vi "Datum_Image_Calibration.vi"(3 "Mode":T11=enum."Run VI", 5 "Traverse line In":T8={"Start X"=1950.0, "Start Y"=0.0, "Start Z"=250.0, "End X"=nan, "End Y"=nan, "End Z"=nan, "No. of pts."=0, "Spacing"=enum."N/A", "Filename"=path "C:/Enflo_Data_Local/2016/EnFlo_Tunnel/Paul_Hayden/Calibrations/Cal_03-2016/50mm_Y_Strip.xls", "Tunnel Speed"=nan, "Averaging time (min)"=nan, "Extra Commands"="", "Carrier_1 Q (l/min)"=nan, "Carrier_2 Q (l/min)"=nan, "Trace Gas Concentration (%)"=nan, "Specific Arguments"="Datum_Image_Calibration.vi; X Fixed", "Comments"="", "Row No"=0, "Row Type Selector"=enum."Run VI Named:", "Completion time"="12:00  22-03-2016", "Row Duration (mins)"=0.08333333333333333, "No. of Valid pts."=0, "Meas Setup File"="Trav_Cam_Picture.xls"} {"Carrier_2 Q (l/min)" format="%#.2f"; "Row Duration (mins)" format="%#.1f"; "Row No" min=0; "Trace Gas Concentration (%)" min=0.0 format="%#_4f"; "Carrier_1 Q (l/min)" format="%#.2f"; "Tunnel Speed" format="%#.2f"; "Start X" format="%#.2f"; "Start Y" format="%#.2f"; "Start Z" format="%#.2f"; "End X" format="%#.2f"; "End Y" format="%#.2f"; "End Z" format="%#.2f"; "Averaging time (min)" min=0.0 format="%#.2f"}) -> (0 "Error Message":string, 1 "Status":T7, 2 "Traverse line Out":T8={"Start X"=1950.0, "Start Y"=0.0, "Start Z"=250.0, "End X"=nan, "End Y"=nan, "End Z"=nan, "No. of pts."=0, "Spacing"=enum."N/A", "Filename"=path "C:/Enflo_Data_Local/2016/EnFlo_Tunnel/Paul_Hayden/Calibrations/Cal_03-2016/50mm_Y_Strip.xls", "Tunnel Speed"=nan, "Averaging time (min)"=nan, "Extra Commands"="", "Carrier_1 Q (l/min)"=nan, "Carrier_2 Q (l/min)"=nan, "Trace Gas Concentration (%)"=nan, "Specific Arguments"="Datum_Image_Calibration.vi; X Fixed", "Comments"="", "Row No"=0, "Row Type Selector"=enum."Run VI Named:", "Completion time"="12:00  22-03-2016", "Row Duration (mins)"=0.08333333333333333, "No. of Valid pts."=0, "Meas Setup File"="Trav_Cam_Picture.xls"} {"Carrier_2 Q (l/min)" format="%#.2f"; "Row Duration (mins)" format="%#.1f"; "Row No" min=0; "Trace Gas Concentration (%)" min=0.0 format="%#_4f"; "Carrier_1 Q (l/min)" format="%#.2f"; "Tunnel Speed" format="%#.2f"; "Start X" format="%#.2f"; "Start Y" format="%#.2f"; "Start Z" format="%#.2f"; "End X" format="%#.2f"; "End Y" format="%#.2f"; "End Z" format="%#.2f"; "Averaging time (min)" min=0.0 format="%#.2f"})   [LabVIEW 2015]
uses:
  Gen Trav/Traverse_cluster.ctl
  Gen Trav/Spacing.ctl
  Controls/Multi_run_mode.ctl
  Controls/User_Specific_mode.ctl
  Gen Trav/Multi_Run_Status.ctl
  Utilities/Image acquisition and processing/Feature detection/Typedefs/ROI bounds.ctl
  Utilities/Image acquisition and processing/Feature detection/Typedefs/Theta range.ctl
  Camera Server/Camera enum/Camera enum.ctl
  Utilities/Image acquisition and processing/Feature detection/Typedefs/Txy range.ctl
  Utilities/Image acquisition and processing/Feature detection/Typedefs/Top level controls.ctl
  Camera Server/Camera enum/Camera resolution.ctl
  Gen Trav/Status_Cluster.ctl
  <vilib>/Analysis/baseanly.llb/Mean (DBL).vi
  Globals/Constants_global.vi
  <vilib>/Analysis/NI_AALBase.lvlib
panel:
  in  "Resolution":T1=2 items=["Low", "Med.", "High", "Max."]
  out "Setup file?":bool
  in  "Controls":T2={"Auto ROI (for rot.)"=FALSE, "Apply scaling"=FALSE, "Apply rotation"=TRUE, "Apply Tx"=FALSE, "Apply Ty"=FALSE, "Keep proc. img"=FALSE}
  in  "Txy range (pixels)":T3={"Tx max (pix)"=150, "Tx min (pix)"=-150, "Ty max (pix)"=10, "Ty min (pix)"=-10}
  in  "Quality":u32=750 max=1000
  in  "Camera":T4="Travcam"
  in  "Theta range (deg)":T5={"theta max (deg)"=20.0, "theta min (deg)"=-20.0}
  in  "ROI to crop (pixels)":T6={"Xmax"=458, "Ymax"=346, "Xmin"=252, "Ymin"=131}
  out "Scale":dbl[](graph)
  out "Angle":dbl[](graph)=[-89.79324776154536, -89.74497086066056, -89.6724887953992, -89.66762827818829]
  out "Displacments":sgl[][](array[numeric])=[[-0.0, -0.0], [-0.0, -5.0], [-0.0, -10.0], [-0.0, 5.0], [-0.0, 10.0]]
  in  "Averaging time (s) (from end)":dbl=1.0
  in  "Duration (s)":dbl=5.0
  # "X           Y            Z"
  # "Start"
  # "End"
  # "X           Y            Z"
  # "Start"
  # "End"
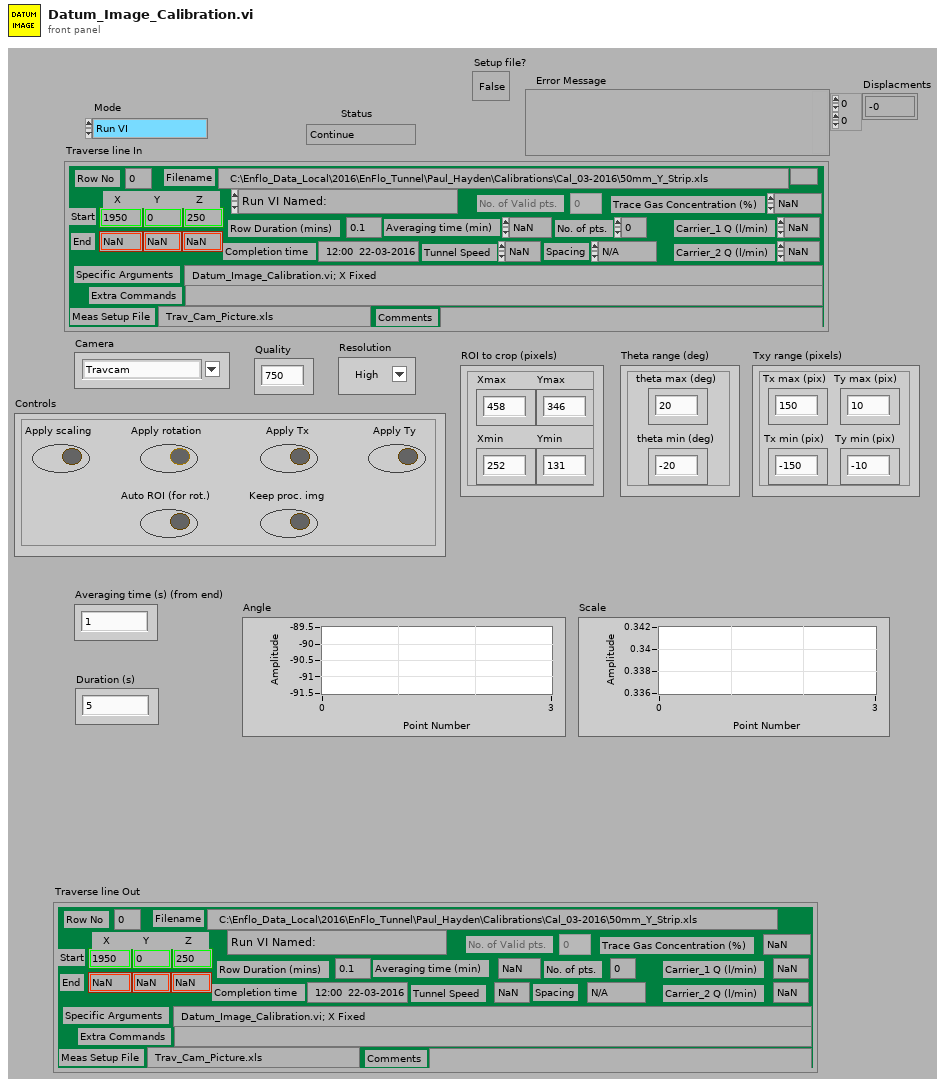
[diagram p1: front panel]
types:
  T1 = typedef "Camera resolution.ctl" = u8
  T2 = typedef "Top level controls.ctl" = cluster{"Auto ROI (for rot.)":bool, "Apply scaling":bool, "Apply rotation":bool, "Apply Tx":bool, "Apply Ty":bool, "Keep proc. img":bool}
  T3 = typedef "Txy range.ctl" = cluster{"Tx max (pix)":i32, "Tx min (pix)":i32, "Ty max (pix)":i32, "Ty min (pix)":i32}
  T4 = typedef "Camera enum.ctl" = string
  T5 = typedef "Theta range.ctl" = cluster{"theta max (deg)":dbl, "theta min (deg)":dbl}
  T6 = typedef "ROI bounds.ctl" = cluster{"Xmax":i32, "Ymax":i32, "Xmin":i32, "Ymin":i32}
  T7 = typedef "Multi_Run_Status.ctl" = enum16{"Continue", "Jump to Next Point", "Jump to Next Row", "Jump To Fall Back", "Terminate Run"}
  T8 = typedef "Traverse_cluster.ctl" = cluster{"Start X":sgl, "Start Y":sgl, "Start Z":sgl, "End X":sgl, "End Y":sgl, "End Z":sgl, "No. of pts.":i32, "Spacing":T9, "Filename":path, "Tunnel Speed":dbl, "Averaging time (min)":dbl, "Extra Commands":string, "Carrier_1 Q (l/min)":dbl, "Carrier_2 Q (l/min)":dbl, "Trace Gas Concentration (%)":dbl, "Specific Arguments":string, "Comments":string, "Row No":i32, "Row Type Selector":T10, "Completion time":string, "Row Duration (mins)":dbl, "No. of Valid pts.":i32, "Meas Setup File":string}
  T9 = typedef "Spacing.ctl" = enum16{"Linear", "Log", "Gauss", "Specified", "N/A"}
  T10 = typedef "Multi_run_mode.ctl" = enum16{"Move Traverse Only", "Set Tunnel Speed Only", "Set Source Only", "Set Measurement Conditions", "Single Measurement", "Vertical Profile", "Lateral Profile", "Longitudinal Profile", "Explore Volume", "Multi-Axis Profile", "Auto Calibrate", "Meas Fast FID Bkgnd", "Check Beam Power", "Scanning Valve Measurement", "Run VI Named:", "Set ADAM Ch", "Wait (minutes)", "Send Message", "Synchronize With:", "Fall Back to this Row", "Turn Off Row Repeating", "Blank Row", "Traverse 3D Volume"}
  T11 = typedef "User_Specific_mode.ctl" = enum16{"Check VI only", "Run VI"}
  T12 = typedef "Status_Cluster.ctl" = cluster{"Status":T7, "Error Type":string, "Error Description":string}
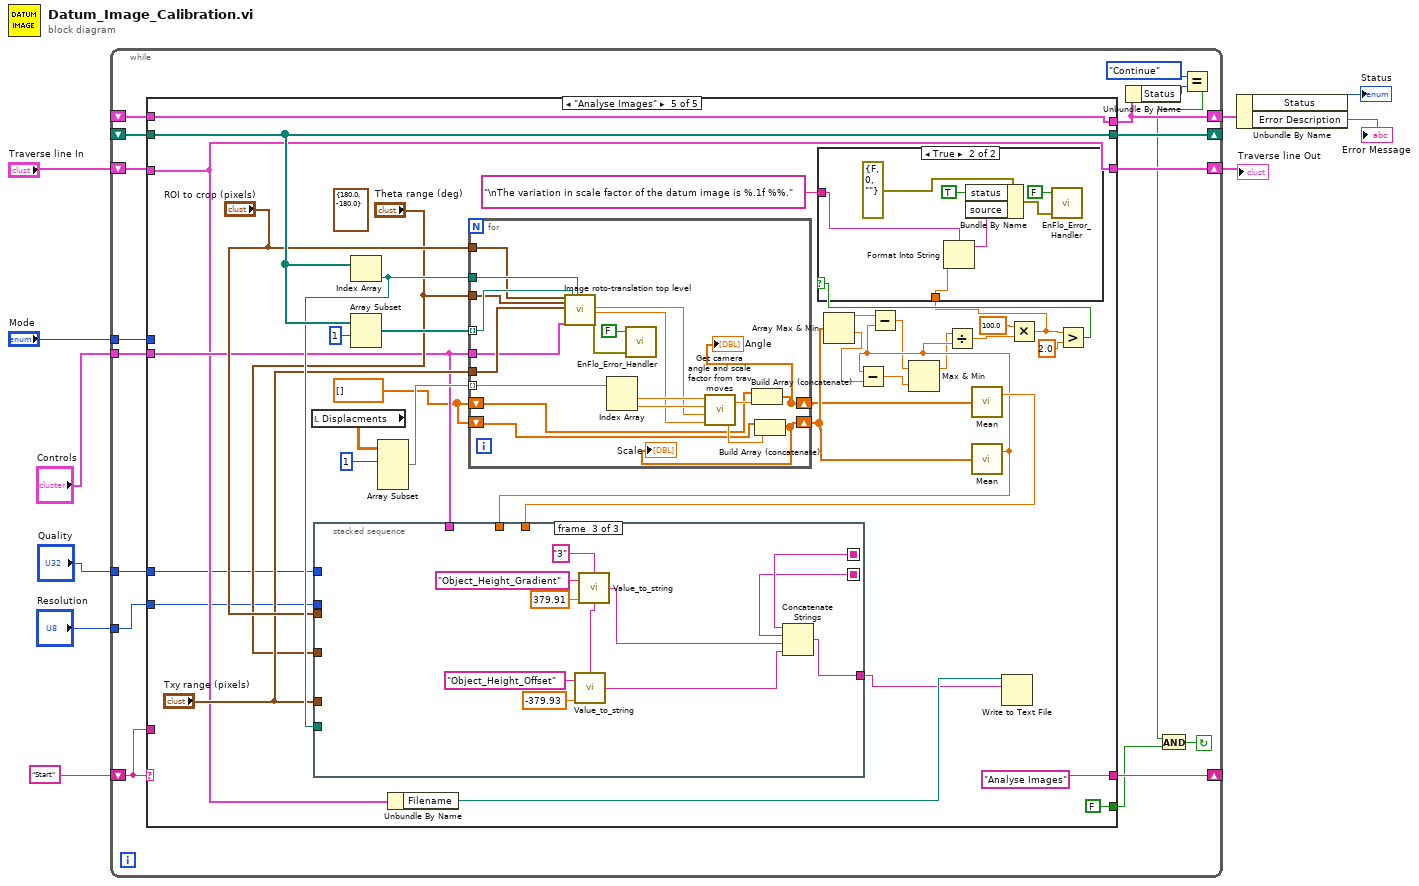
[diagram p0: block diagram]
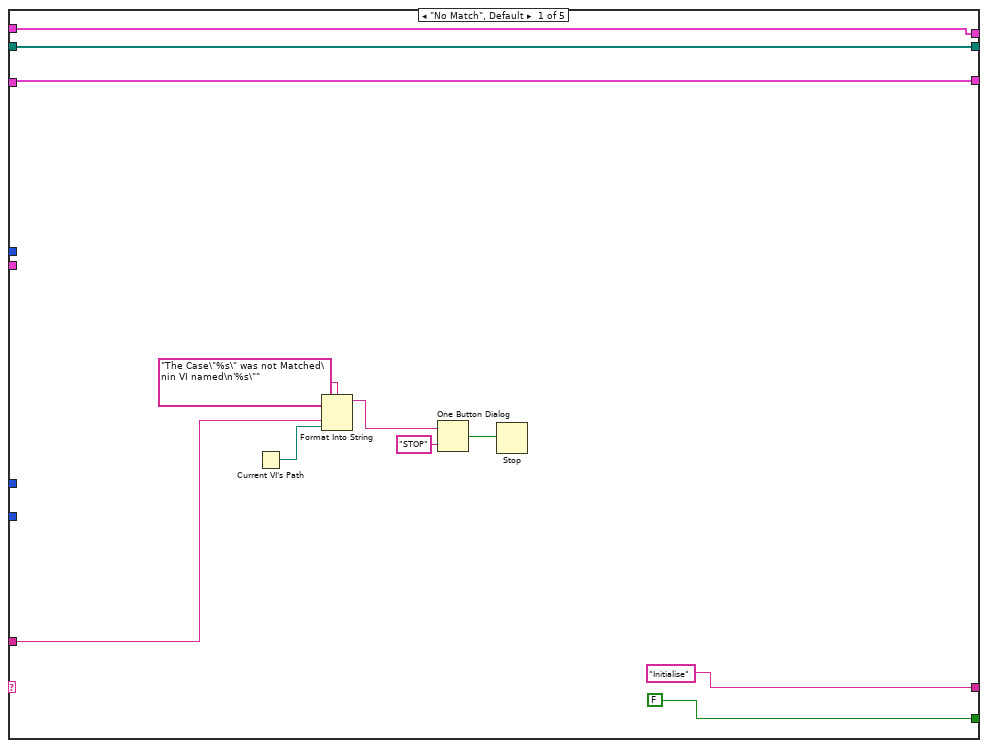
[diagram p2: hidden frame]
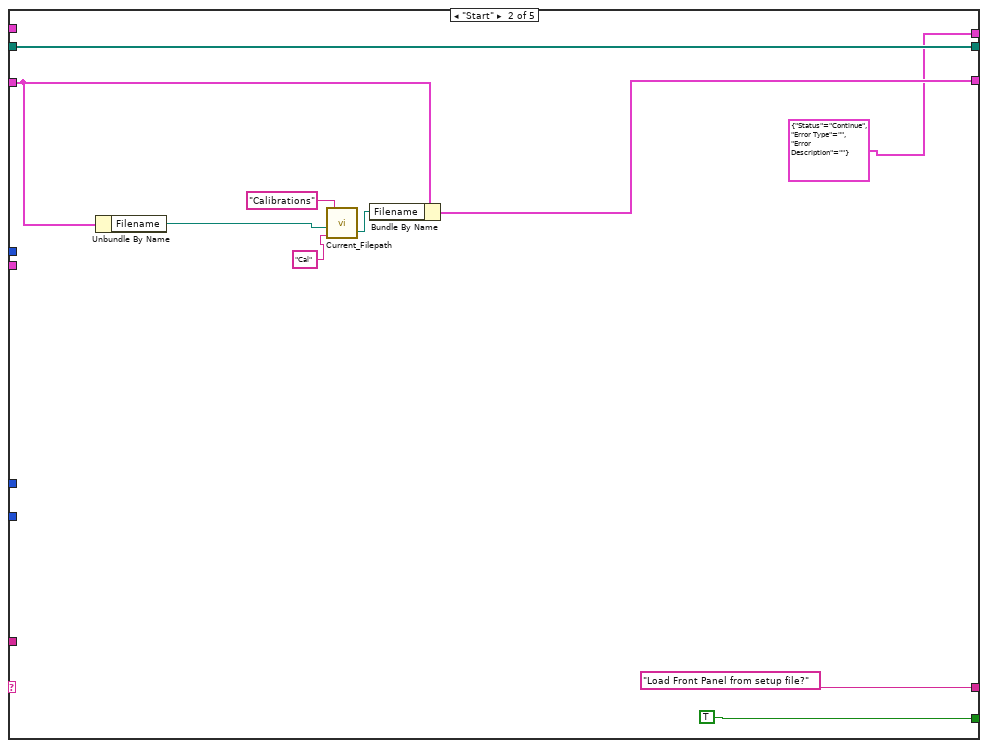
[diagram p3: hidden frame]
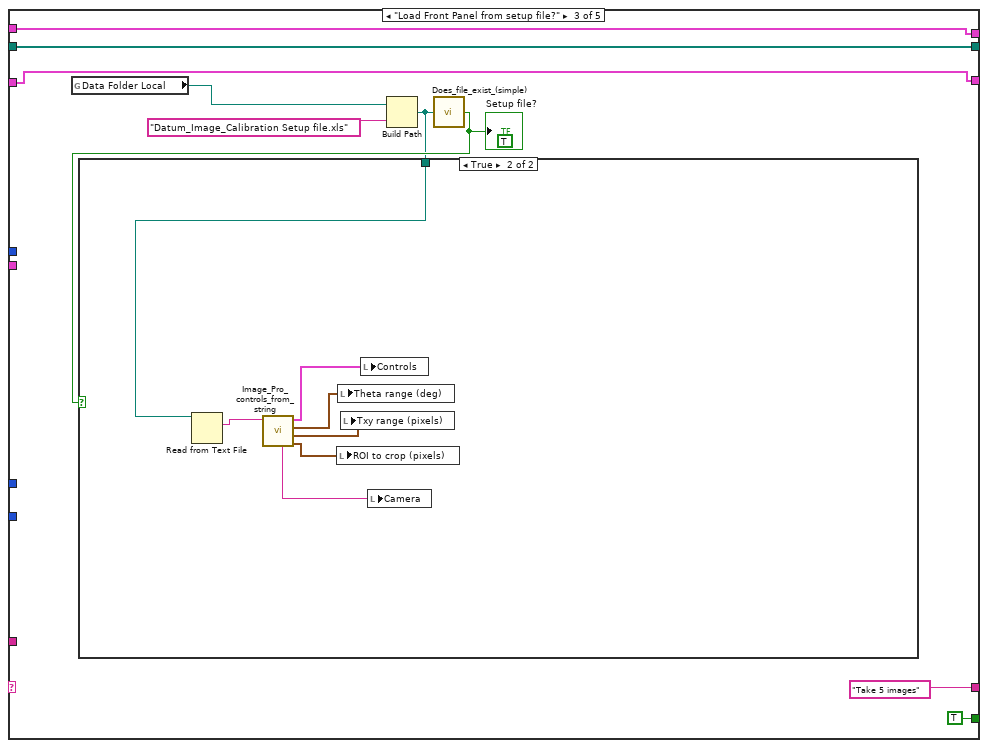
[diagram p4: hidden frame]
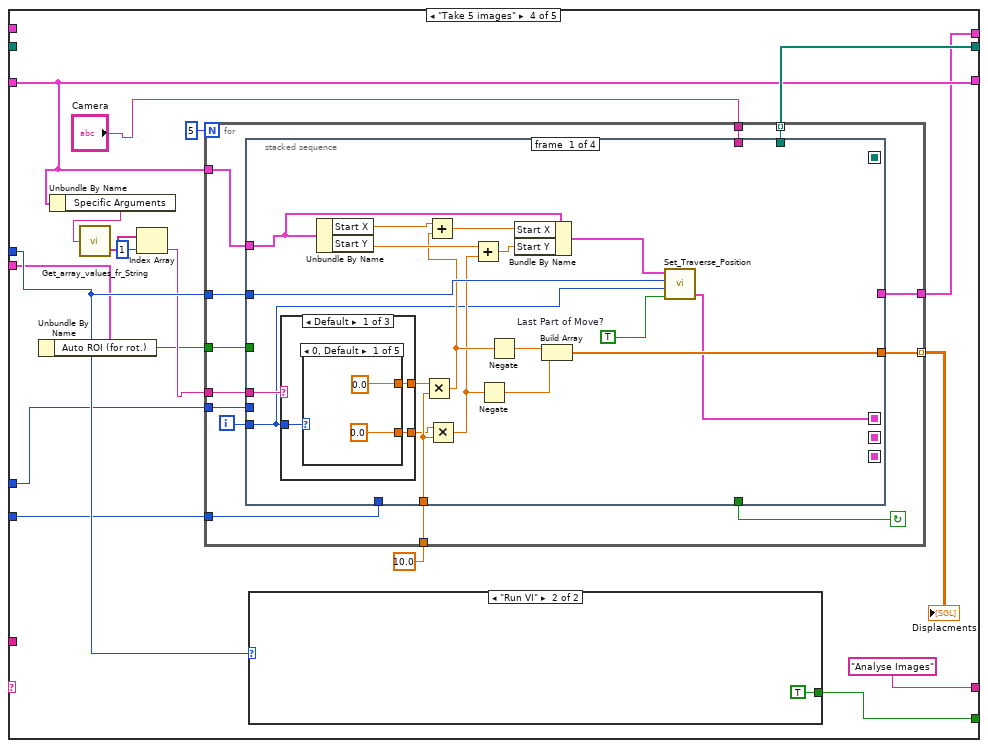
[diagram p6: hidden frame]
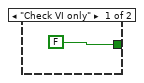
[diagram p7: hidden frame]
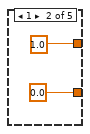
[diagram p8: hidden frame]
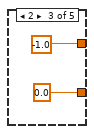
[diagram p9: hidden frame]
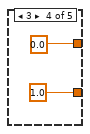
[diagram p10: hidden frame]
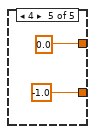
[diagram p11: hidden frame]
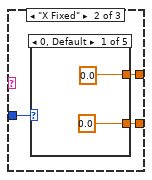
[diagram p12: hidden frame]
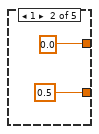
[diagram p13: hidden frame]
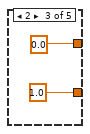
[diagram p14: hidden frame]
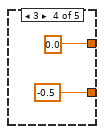
[diagram p15: hidden frame]
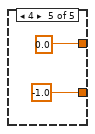
[diagram p16: hidden frame]
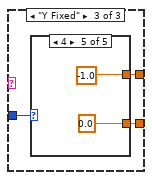
[diagram p17: hidden frame]
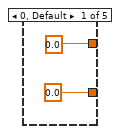
[diagram p18: hidden frame]
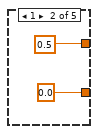
[diagram p19: hidden frame]
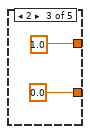
[diagram p20: hidden frame]
diagram:
  n1 = while {
    shift-left: "Start" -> [w26]
    shift-right: [w27] -> _
    tunnel: "Mode" -> [w25]
    shift-right: [w23] -> w7
    shift-left: "Traverse line In" -> [w24]
    shift-right: [w22] -> _
    shift-left: _ -> [w21]
    tunnel: "Controls" -> [w20]
    shift-right: [w19] -> w5
    shift-left: _ -> [w13]
    tunnel: "Quality" -> [w12]
    tunnel: "Resolution" -> [w11]
    stop <- w15 continue-if-true
    n2 = case shown="\"Analyse Images\"" w26 {
      tunnel: [FALSE TRUE TRUE w77 FALSE] -> w16
      tunnel: ["Initialise" "Load Front Panel from setup file?" "Take 5 images" "Analyse Images" "Analyse Images"] -> w27
      tunnel: w26 -> [w33 _ _ _ _]
      tunnel: w25 -> [_ _ _ w78 _]
      tunnel: w24 -> [w30 w43 w50 w70 w225]
      tunnel: [w30 w42 w50 w70 w225] -> w23
      tunnel: [w29 w41 w51 w79 w241] -> w22
      tunnel: w21 -> [w29 w41 w51 _ w241]
      tunnel: w20 -> [_ _ _ w67 w228]
      tunnel: [w28 T12 {"Status"=enum."Continue", "Error Type"="", "Error Description"=""} ("Status Cluster Out") w49 w69 w210] -> w19
      tunnel: w13 -> [w28 _ w49 _ w210]
      tunnel: w12 -> [_ _ _ w68 w211]
      tunnel: w11 -> [_ _ _ w65 w209]
      frame "No Match", Default {
        n3 = Current VI's Path() -> (path=w32:path)
        n4 = Format Into String(format string="The Case\"%s\" was not Matched\nin VI named\n'%s\"" ("Format String"), w33, w32) -> (resulting string=w36:string)  [unwired: 2 in, 1 out]
        n5 = One Button Dialog(message=w36, button name ("OK")="STOP") -> (true=w34:bool)
        n6 = Stop(stop? (T)=w34) -> ()
      }
      frame "Start" {
        n7 = Unbundle By Name(w43) -> ("Filename"=w45:path)
        n8 = call "Current_Filepath.vi"("Short_Name"="Cal" ("Data Type"), "Filename in"=w45, "Data Type"="Calibrations") -> ("Filename Out"=w40:path)  [unwired: 1 in, 1 out]
        n9 = Bundle By Name(cluster=w43, "Filename"=w40) -> (w42:T8)
      }
      frame "Load Front Panel from setup file?" {
        (unwired) TRUE ("exists?")
        n10 = global read "Constants_global.vi" "Data Folder Local"() -> (w55:path)
        n11 = Build Path(base path=w55, name or relative path="Datum_Image_Calibration Setup file.xls") -> (appended path=w52:path)
        n12 = call "Does_file_exist_(simple).vi"("Pathname"=w52) -> ("exists?"=w53:bool)
        "Setup file?" <- w53
        n13 = case shown="True" w53 {
          tunnel: w52 -> [_ w64]
          frame False {
          }
          frame True {
            n14 = Read from Text File(file (use dialog)=w64) -> (text=w63:string)  [unwired: 3 in, 3 out]
            n15 = call "Image_Pro_controls_from_string.vi"("Setup String"=w63) -> ("ROI to crop (pixels)"=w59:T6, "Txy range (pixels)"=w60:T3, "Theta range (deg)"=w61:T5, "Controls"=w62:T2, "Camera"=w58:string)  [unwired: 4 in, 2 out]
            n16 = local write "ROI to crop (pixels)"(w59) -> ()
            n17 = local write "Theta range (deg)"(w61) -> ()
            n18 = local write "Txy range (pixels)"(w60) -> ()
            n19 = local write "Controls"(w62) -> ()
            n20 = local write "Camera"(w58) -> ()
          }
        }
      }
      frame "Take 5 images" {
        n21 = Unbundle By Name(w67) -> ("Auto ROI (for rot.)"=w66:bool)
        n22 = Unbundle By Name(w70) -> ("Specific Arguments"=w75:string)
        n23 = call "Get_array_values_fr_String.vi"("String Value"=w75) -> ("String array"=w74:string[])  [unwired: 1 out]
        n24 = Index Array(array=w74, index=1) -> (element=w72:string)
        n25 = for {
          N: 5 -> [_]
          tunnel: w70 -> [w97]
          tunnel: w78 -> [w96]
          tunnel: sgl 10.0 ("y") -> [w94]
          tunnel: [w93] -> w79 mode=indexing
          tunnel: [w92] -> w76 mode=indexing
          tunnel: w72 -> [w91]
          tunnel: "Camera" -> [w90]
          tunnel: [w88] -> w69
          tunnel: w68 -> [w87]
          tunnel: w66 -> [w86]
          tunnel: w65 -> [w85]
          i -> [w95]
          stop <- w89 continue-if-true
          n26 = stacked-sequence {
            seq-local: [_ w160 _ _] -> [_ _ w189 _]
            seq-local: [w98 _ _ _] -> [_ w158 w187 w208]
            seq-local: [_ w159 _ _] -> [_ _ _ w207]
            seq-local: [_ _ w188 _] -> [_ _ _ w205]
            tunnel: w97 -> [w108 w163 _ _]
            tunnel: w96 -> [w116 w162 w185 _]
            tunnel: w95 -> [w100 _ w192 _]
            tunnel: w94 -> [w113 _ _ _]
            tunnel: [_ w160 _ _] -> w93
            tunnel: [w104 _ _ _] -> w92
            tunnel: w91 -> [w101 _ _ _]
            tunnel: w90 -> [_ w161 _ _]
            tunnel: [_ _ _ w203] -> w89
            tunnel: [_ _ _ w201] -> w88
            tunnel: w87 -> [_ w157 _ _]
            tunnel: w86 -> [_ _ w183 _]
            tunnel: w85 -> [_ w156 _ _]
            frame #0 {
              w99 = TRUE  # Last Part of Move?
              n27 = case shown="Default" w101 {
                tunnel: w100 -> [w119 w132 w145]
                tunnel: [w118 w131 w144] -> w114
                tunnel: [w117 w130 w143] -> w112
                frame Default {
                  n28 = case shown="0, Default" w119 {
                    tunnel: [sgl 0.0 ("Start Y") sgl 1.0 ("Start Y") sgl -1.0 ("Start Y") sgl 0.0 ("Start Y") sgl 0.0 ("Start Y")] -> w118
                    tunnel: [sgl 0.0 ("Start Y") sgl 0.0 ("Start Y") sgl 0.0 ("Start Y") sgl 1.0 ("Start Y") sgl -1.0 ("Start Y")] -> w117
                    frame 0, Default {
                    }
                    frame 1 {
                    }
                    frame 2 {
                    }
                    frame 3 {
                    }
                    frame 4 {
                    }
                  }
                }
                frame "X Fixed" {
                  n29 = case shown="0, Default" w132 {
                    tunnel: [sgl 0.0 ("Start Y") sgl 0.0 ("Start Y") sgl 0.0 ("Start Y") sgl 0.0 ("Start Y") sgl 0.0 ("Start Y")] -> w131
                    tunnel: [sgl 0.0 ("Start Y") sgl 0.5 ("Start Y") sgl 1.0 ("Start Y") sgl -0.5 ("Start Y") sgl -1.0 ("Start Y")] -> w130
                    frame 0, Default {
                    }
                    frame 1 {
                    }
                    frame 2 {
                    }
                    frame 3 {
                    }
                    frame 4 {
                    }
                  }
                }
                frame "Y Fixed" {
                  n30 = case shown="4" w145 {
                    tunnel: [sgl 0.0 ("Start Y") sgl 0.5 ("Start Y") sgl 1.0 ("Start Y") sgl -0.5 ("Start Y") sgl -1.0 ("Start Y")] -> w144
                    tunnel: [sgl 0.0 ("Start Y") sgl 0.0 ("Start Y") sgl 0.0 ("Start Y") sgl 0.0 ("Start Y") sgl 0.0 ("Start Y")] -> w143
                    frame 0, Default {
                    }
                    frame 1 {
                    }
                    frame 2 {
                    }
                    frame 3 {
                    }
                    frame 4 {
                    }
                  }
                }
              }
              n31 = Unbundle By Name(w108) -> ("Start X"=w115:sgl, "Start Y"=w111:sgl)
              n32 = Multiply(x=w114, y=w113) -> (x*y=w106:sgl)
              n33 = Add(x=w115, y=w106) -> (x+y=w107:sgl)
              n34 = Multiply(x=w112, y=w113) -> (x*y=w105:sgl)
              n35 = Add(x=w111, y=w105) -> (x+y=w110:sgl)
              n36 = Negate(x=w105) -> (-x=w102:sgl)
              n37 = Negate(x=w106) -> (-x=w103:sgl)
              n38 = Bundle By Name(cluster=w108, "Start X"=w107, "Start Y"=w110) -> (w109:T8)
              n39 = Build Array(w103, w102) -> (w104:sgl[])
              n40 = call "Set_Traverse_Position.vi"("Last Part of Move?"=w99, "Currently on Point"=w100, "Simulate/Run"=w116, "Traverse line"=w109) -> ("Status Cluster"=w98:T12)  [unwired: 2 in]
            }
            frame #1 {
              n41 = case shown="\"Run VI\"" w162 {
                tunnel: w163 -> [_ w178]
                tunnel: [path "" ("stripped path") w172] -> w160
                tunnel: w161 -> [_ w171]
                tunnel: [w164 w168] -> w159
                tunnel: w158 -> [w164 _]
                tunnel: w157 -> [_ w167]
                tunnel: w156 -> [_ w166]
                frame "Check VI only" {
                }
                frame "Run VI" {
                  n42 = Unbundle By Name(w178) -> ("Filename"=w175:path)
                  n43 = call "Get_Data_Base_file_code.vi"("Data Type"="Raw_Calibrations", "Results Filename"=w175, "Short_Name"="Raw_Cal" ("Data Type")) -> ("Raw Data File Name"=w173:path)  [unwired: 1 in, 3 out]
                  n44 = Strip Path(path=w173) -> (stripped path=w174:path, name=w177:string)
                  n45 = call "Add_filename_suffix.vi"("Filename"=w177) -> ("Base name"=w176:string)  [unwired: 1 in, 3 out]
                  n46 = call "Async Get averaged image from CamServer and display locally.vi"("Quality"=w167, "Resolution"=w166, "Camera"=w171, "Averaging time (s) (from end)"="Averaging time (s) (from end)", "Duration (s)"="Duration (s)", "Image directory path"=w174, "Image name"=w176) -> ("Error out"=w170:errorcluster, "Image file path"=w172:path)  [unwired: 3 in]
                  n47 = call "Error_to_Status_Cluster.vi"("Error In"=w170, "Status"=Multi_Run_Status."Terminate Run") -> ("Status Cluster Out"=w168:T12)
                }
              }
            }
            frame #2 {
              n48 = Equal To 0?(x=w192) -> (x = 0?=w191:bool)
              n49 = Equal?(x=User_Specific_mode."Run VI" ("Mode"), y=w185) -> (x = y?=w184:bool)
              n50 = Compound Arithmetic op=AND(w184, invert w183, w191) -> (w190:bool)
              n51 = case shown="True" w190 {
                tunnel: w189 -> [_ w199]
                tunnel: [w193 w195] -> w188
                tunnel: w187 -> [w193 _]
                frame False {
                }
                frame True {
                  n52 = call "Draw ROI (user interactive).vi"("Dialog title message"="Please draw your region of interest rectangle", "Image file path"=w199) -> ("Error out"=w197:errorcluster, "ROI to crop (pixels)"=w198:T6)
                  n53 = case shown="Error" w197 {
                    tunnel: w198 -> [w200 _]
                    frame No Error {
                      n54 = local write "ROI to crop (pixels)"(w200) -> ()
                    }
                    frame Error {
                    }
                  }
                  n55 = call "Error_to_Status_Cluster.vi"("Error In"=w197, "Status"=Multi_Run_Status."Terminate Run") -> ("Status Cluster Out"=w195:T12)
                }
              }
            }
            frame #3 {
              n56 = call "Merge_Status_Clusters.vi"("Status Cluster 2"=w207, "Status Cluster 1"=w208) -> ("Status Cluster Out"=w206:T12)
              n57 = call "Merge_Status_Clusters.vi"("Status Cluster 2"=w205, "Status Cluster 1"=w206) -> ("Status Cluster Out"=w201:T12)
              n58 = Unbundle By Name(w201) -> ("Status"=w202:T7)
              n59 = Equal?(x=Multi_Run_Status."Continue" ("Status"), y=w202) -> (x = y?=w203:bool)
            }
          }
        }
        "Displacments" <- w76
        n60 = case shown="\"Run VI\"" w78 {
          tunnel: [FALSE TRUE] -> w77
          frame "Check VI only" {
          }
          frame "Run VI" {
          }
        }
      }
      frame "Analyse Images" {
        w212 = dbl[] []
        (unwired) T5 {"theta max (deg)"=180.0, "theta min (deg)"=-180.0} ("Theta range (deg)")
        n61 = local read "Displacments"() -> (w239:sgl[][])
        n62 = Index Array(array=w241) -> (element=w235:path)  [unwired: 1 in]
        n63 = Array Subset(array=w241, index=1) -> (w237:path[])  [unwired: 1 in]
        n64 = Array Subset(array=w239, index (row)=1 ("index")) -> (w238:sgl[][])  [unwired: 3 in]
        n65 = Unbundle By Name(w225) -> ("Filename"=w234:path)
        n66 = for {
          tunnel: w238 -> [w299] mode=indexing
          tunnel: w235 -> [w296]
          tunnel: w237 -> [w295] mode=indexing
          tunnel: "ROI to crop (pixels)" -> [w294]
          tunnel: "Txy range (pixels)" -> [w291]
          tunnel: "Theta range (deg)" -> [w290]
          tunnel: w228 -> [w287]
          shift-right: [w282] -> w216
          shift-left: w212 -> [w283]
          shift-right: [w281] -> w217
          shift-left: w212 -> [w284]
          n67 = call "Image roto-translation top level.vi"("ROI to crop (pixels)"=w294, "Theta range (deg)"=w290, "Txy range (pixels)"=w291, "Controls"=w287, "Test image file path"=w295, "Reference image file path"=w296) -> ("Tx (pixels)"=w289:dbl, "Ty (pixels)"=w288:dbl, "Error Out"=w292:errorcluster)  [unwired: 7 in, 4 out]
          n68 = Index Array(array=w299) -> (element #1=w298:sgl, element #2=w297:sgl)  [unwired: 2 in]
          n69 = call "EnFlo_Error_Handler.vi"("error in (no error)"=w292, "Dialog Box (T)"=FALSE) -> ()  [unwired: 1 in, 3 out]
          n70 = call "Get camera angle and scale factor from trav moves.vi"("dy (pix)"=w288, "dx (pix)"=w289, "dy (mm)"=w297, "dx (mm)"=w298) -> ("scale factor (mm / pixel)"=w285:dbl, "camera angle, ccw+ rel. to trav. (deg)"=w286:dbl)
          n71 = Build Array (concatenate)(w283, w286) -> (w282:dbl[])
          "Angle" <- w282
          n72 = Build Array (concatenate)(w284, w285) -> (w281:dbl[])
          "Scale" <- w281
        }
        n73 = Array Max & Min(array=w217) -> (max value=w220:dbl, min value=w218:dbl)  [unwired: 2 out]
        n74 = call-poly <vilib>:"Mean.vi"("X"=w216) -> ("mean"=w233:dbl)  [unwired: 1 out]
        n75 = call-poly <vilib>:"Mean.vi"("X"=w217) -> ("mean"=w219:dbl)  [unwired: 1 out]
        n76 = stacked-sequence {
          seq-local: [w253 _ _] -> [_ _ w279]
          seq-local: [_ w265 _] -> [_ _ w278]
          tunnel: w235 -> [w259 _ _]
          tunnel: w233 -> [w254 _ _]
          tunnel: w219 -> [w252 _ _]
          tunnel: "ROI to crop (pixels)" -> [_ w269 _]
          tunnel: [_ _ w280] -> w231
          tunnel: "Theta range (deg)" -> [_ w268 _]
          tunnel: "Txy range (pixels)" -> [_ w267 _]
          tunnel: w228 -> [_ w270 _]
          tunnel: w211 -> [_ w264 _]
          tunnel: w209 -> [_ w263 _]
          frame #0 {
            n77 = call "Path_2_String.vi"("Real Path"=w259) -> ("Path String"=w260:string)
            n78 = call "Value_to_string.vi"("Value"=w254, "Label for value"="Camera Angle") -> ("Output string"=w256:string)  [unwired: 1 in]
            n79 = call "Date_and_Time_to_string.vi"() -> ("Date and time (spreadsheet)"=w255:string)
            n80 = call "Value_to_string.vi"("Value"=w252, "Label for value"="scale factor (mm / pixel)") -> ("Output string"=w257:string)  [unwired: 1 in]
            n81 = call "Characters_to_string.vi"("Characters to write"=w260, "Label for characters"="Datum Image Filename") -> ("Output string"=w251:string)
            n82 = Concatenate Strings(w255, w256, w257, w251) -> (w253:string)
          }
          frame #1 {
            n83 = local read "Camera"() -> (w266:T4)
            n84 = call "Image_Pro_controls_to_string.vi"("Quality"=w264, "Camera"=w266, "Resolution"=w263, "ROI to crop (pixels)"=w269, "Txy range (pixels)"=w267, "Theta range (deg)"=w268, "Controls"=w270) -> ("Setup String"=w265:string)  [unwired: 4 in]
          }
          frame #2 {
            w271 = "3" ("precision")
            n85 = call "Value_to_string.vi"("precision"=w271, "Value"=-379.93, "Label for value"="Object_Height_Offset") -> ("Output string"=w272:string)
            n86 = call "Value_to_string.vi"("precision"=w271, "Value"=379.91, "Label for value"="Object_Height_Gradient") -> ("Output string"=w273:string)
            n87 = Concatenate Strings(w279, w278, w273, w272) -> (w280:string)
          }
        }
        n88 = Subtract(x=w219, y=w218) -> (x-y=w214:dbl)
        n89 = Subtract(x=w220, y=w219) -> (x-y=w215:dbl)
        n90 = Max & Min(x=w215, y=w214) -> (max(x,y)=w213:dbl)  [unwired: 1 out]
        n91 = Divide(x=w213, y=w219) -> (x/y=w224:dbl)
        n92 = Write to Text File(file (use dialog)=w234, text=w231) -> ()  [unwired: 2 in, 3 out]
        n93 = Multiply(x=100.0, y=w224) -> (x*y=w222:dbl)
        n94 = Greater?(x=w222, y=2.0) -> (0:w226:bool)
        n95 = case shown="True" w226 {
          tunnel: w222 -> [_ w250]
          tunnel: "\nThe variation in scale factor of the datum image is %.1f %%." ("format string") -> [_ w249]
          frame False {
          }
          frame True {
            n96 = Format Into String(format string=w249, w250) -> (resulting string=w246:string)  [unwired: 2 in, 1 out]
            n97 = Bundle By Name(cluster=errorcluster {"status"=FALSE, "code"=0, "source"=""} ("error in (no error)"), "status"=TRUE, "source"=w246) -> (w244:errorcluster)
            n98 = call "EnFlo_Error_Handler.vi"("error in (no error)"=w244, "Dialog Box (T)"=FALSE) -> ()  [unwired: 1 in, 3 out]
          }
        }
      }
    }
    n99 = Unbundle By Name(w19) -> ("Status"=w18:T7)
    n100 = Equal?(x=Multi_Run_Status."Continue" ("Status"), y=w18) -> (x = y?=w14:bool)
    n101 = And(x=w14, y=w16) -> (x .and. y?=w15:bool)
  }
  "Traverse line Out" <- w7
  n102 = Unbundle By Name(w5) -> ("Status"=→"Status":T7, "Error Description"=→"Error Message":string)
